vi "Missing Property Error.vi"(8 "error in (no error)":errorcluster, 10 "Property Name":string, 11 "Hardware Ref in":T1 format="%.0x") -> (0 "error out":errorcluster, 3 "Hardware Ref out":T1 format="%.0x")   [LabVIEW 2017, in "Routing and Faulting Hardware API.lvlib"]
uses:
  Routing and Faulting Hardware API.lvlib
  <vilib>/NI Veristand/Custom Device API/Custom Device Item Ref.ctl
  <vilib>/NI Veristand/Custom Device API/Custom Device API.lvlib
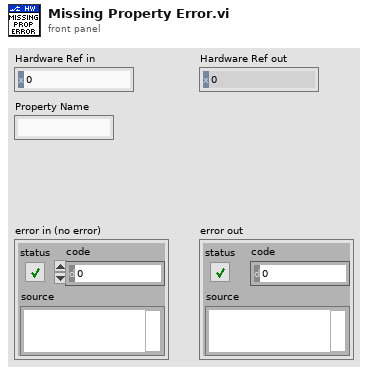
[diagram p1: front panel]
types:
  T1 = typedef "Custom Device API.lvlib/Custom Device Item Ref.ctl" = u64
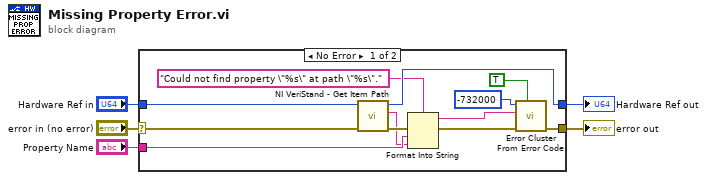
[diagram p0: block diagram]
diagram:
  n1 = case shown="No Error" "error in (no error)" {
    selector: "error in (no error)" -> [w13 w19]
    tunnel: "Property Name" -> [w17 _]
    tunnel: [w16 w18] -> w4
    tunnel: "Hardware Ref in" -> [w15 w18]
    tunnel: [w14 w19] -> w2
    frame No Error {
      n2 = call <vilib>:"NI VeriStand - Get Item Path.vi"("error in (no error)"=w13, "Item Ref in"=w15) -> ("error out"=w11:errorcluster, "Path"=w9:string, "Item Ref out"=w16:T1)  [unwired: 6 in, 1 out]
      n3 = Format Into String(format string="Could not find property \"%s\" at path \"%s\"." ("error message (\"\")"), error in=w11, w17, w9) -> (resulting string=w12:string, error out=w10:errorcluster)  [unwired: 1 in]
      n4 = call <vilib>:"Error Cluster From Error Code.vi"("show call chain? (False)"=TRUE, "error in (no error)"=w10, "error message (\"\")"=w12, "error code (0)"=-732000) -> ("error out"=w14:errorcluster)  [unwired: 5 in]
    }
    frame Error {
    }
  }
  "Hardware Ref out" <- w4
  "error out" <- w2
